vi "Parse ExptParam.vi"(8 "error in (no error)":errorcluster, 11 "params in":variant) -> (0 "error out":errorcluster, 2 "value":variant, 3 "key":string)   [LabVIEW 2019, in "Inst.Transport.lvclass"]
uses:
  Inst.Transport.lvclass
  <vilib>/JDP Science/JSONtext/JSONtext.lvlib
  <vilib>/PRIrvin/JSON-RPC/JSON-RPC.lvlib
panel:
  in  "history":string
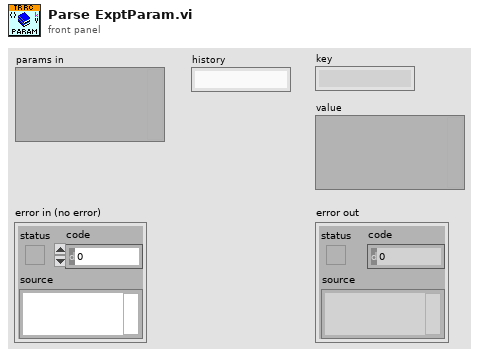
[diagram p1: front panel]
types:
  T1 = typedef "JSONtext.lvlib/JSON Value Type.ctl" = enum16{"Not a JSON Value", "JSON Object", "JSON Array", "String", "Number", "true", "false", "null"}
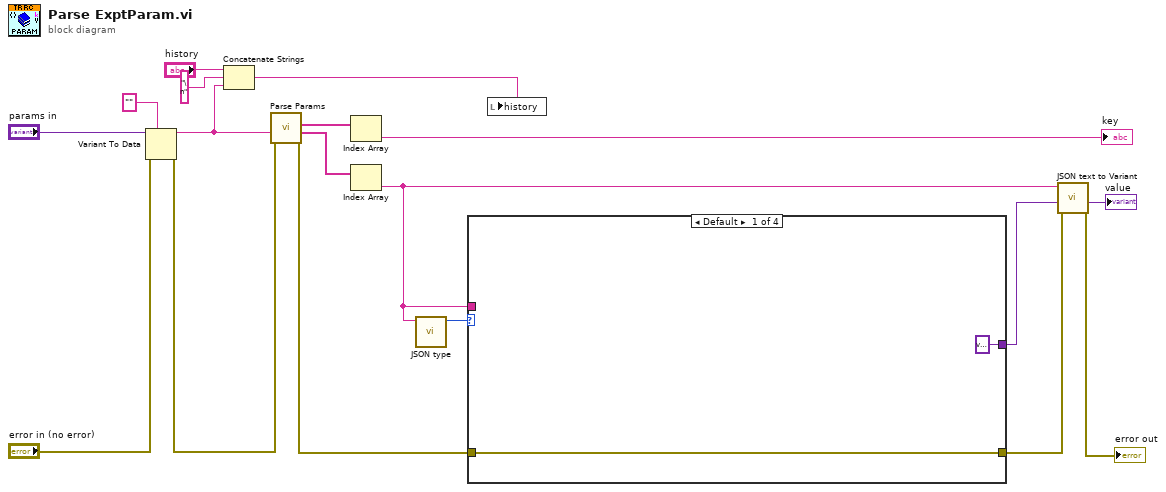
[diagram p0: block diagram]
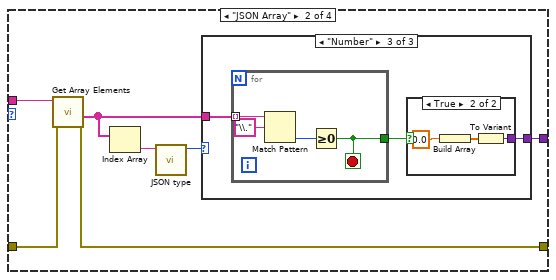
[diagram p2: hidden frame]
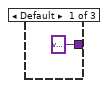
[diagram p3: hidden frame]
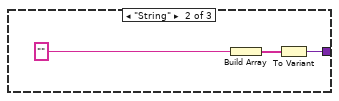
[diagram p4: hidden frame]
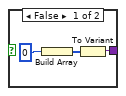
[diagram p5: hidden frame]
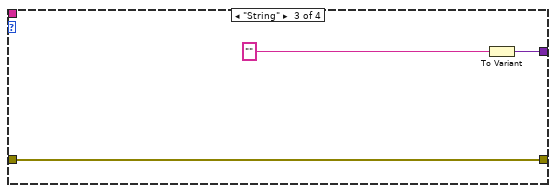
[diagram p6: hidden frame]
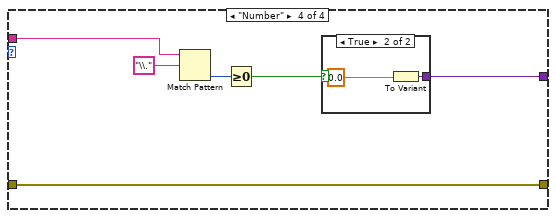
[diagram p7: hidden frame]
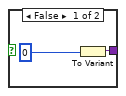
[diagram p8: hidden frame]
diagram:
  n1 = Variant To Data(error in="error in (no error)", type="", Variant="params in") -> (data=w2:string, error out=w6:errorcluster)
  n2 = Concatenate Strings("history", "\n" ("string"), w2) -> (w1:string)
  n3 = call <vilib>:"Parse Params.vi"("error in (no error)"=w6, "<JSON> Params"=w2) -> ("error out"=w12:errorcluster, "Params"=w9:string[], "Names"=w17:string[])  [unwired: 7 in]
  n4 = Index Array(array=w17) -> (element=→"key":string)  [unwired: 1 in]
  n5 = Index Array(array=w9) -> (element=w14:string)  [unwired: 1 in]
  n6 = call <vilib>:"JSON type.vi"("JSON"=w14) -> ("JSON Value Type"=w13:T1)  [unwired: 9 in, 1 out]
  n7 = case shown="Default" w13 {
    tunnel: w14 -> [_ w27 _ w51]
    tunnel: [variant ("Variant") w24 w47 w52] -> w15
    tunnel: w12 -> [w19 w22 w45 w48]
    tunnel: [w19 w21 w45 w48] -> w11
    frame Default {
    }
    frame "JSON Array" {
      n8 = call <vilib>:"Get Array Elements.vi"("error in (no error)"=w22, "JSON"=w27) -> ("error out"=w21:errorcluster, "<JSON>"=w23:string[])  [unwired: 7 in, 1 out]
      n9 = Index Array(array=w23) -> (element=w26:string)  [unwired: 1 in]
      n10 = call <vilib>:"JSON type.vi"("JSON"=w26) -> ("JSON Value Type"=w25:T1)  [unwired: 9 in, 1 out]
      n11 = case shown="\"Number\"" w25 {
        tunnel: [variant ("Variant") w29 w34] -> w24
        tunnel: w23 -> [_ _ w33]
        frame Default {
        }
        frame "String" {
          n12 = Build Array("") -> (w30:string[])
          n13 = To Variant(anything=w30) -> (Variant=w29:variant)
        }
        frame "Number" {
          n14 = for {
            tunnel: w33 -> [w44] mode=indexing
            tunnel: [w41] -> w32
            stop <- w41 stop-if-true
            n15 = Match Pattern(string=w44, regular expression="\\.") -> (offset past match=w42:i32)  [unwired: 1 in, 3 out]
            n16 = Greater Or Equal To 0?(x=w42) -> (x >= 0?=w41:bool)
          }
          n17 = case shown="True" w32 {
            tunnel: [w35 w39] -> w34
            frame False {
              n18 = Build Array(0) -> (w36:i32[])
              n19 = To Variant(anything=w36) -> (Variant=w35:variant)
            }
            frame True {
              n20 = Build Array(0.0) -> (w40:dbl[])
              n21 = To Variant(anything=w40) -> (Variant=w39:variant)
            }
          }
        }
      }
    }
    frame "String" {
      n22 = To Variant(anything="") -> (Variant=w47:variant)
    }
    frame "Number" {
      n23 = Match Pattern(string=w51, regular expression="\\.") -> (offset past match=w49:i32)  [unwired: 1 in, 3 out]
      n24 = Greater Or Equal To 0?(x=w49) -> (x >= 0?=w53:bool)
      n25 = case shown="True" w53 {
        tunnel: [w55 w57] -> w52
        frame False {
          n26 = To Variant(anything=0) -> (Variant=w55:variant)
        }
        frame True {
          n27 = To Variant(anything=0.0) -> (Variant=w57:variant)
        }
      }
    }
  }
  n28 = local write "history"(w1) -> ()
  n29 = call <vilib>:"JSON text to Variant.vi"("error in (no error)"=w11, "Data Type"=w15, "JSON"=w14) -> ("error out"=→"error out":errorcluster, "Variant out"=→"value":variant)  [unwired: 7 in]
